vi "Relay Experiment V2 - Ramps.vi"() -> ()   [LabVIEW 2020]
uses:
  <vilib>/Analysis/1siggen.llb/Ramp Pattern by Samples.vi
  <vilib>/DAQmx/write.llb/DAQmx Write (Analog 1D Wfm NChan NSamp).vi
  <vilib>/DAQmx/create/channels.llb/DAQmx Create Channel (AO-Voltage-Basic).vi
  <vilib>/DAQmx/configure/timing.llb/DAQmx Timing (Use Waveform).vi
  <vilib>/DAQmx/miscellaneous.llb/DAQmx Fill In Error Info.vi
  <vilib>/Analysis/NI_AALBase.lvlib
  <vilib>/measure/NI_MABase.lvlib
panel:
  in  "Trigger 2 Channel":tag="Dev2/ao3"
  in  "AC Output Channel":tag="Dev2/ao1"
  in  "Trigger 1 Channel":tag="Dev2/ao2"
  in  "DC Output Channel":tag="Dev2/ao0"
  out "DC Sampling\nFrequency (Hz)":dbl
  in  "Stop":bool
  in  "DC-to-AC\nDelay Time (ms)":dbl min=0.0 step=1.0
  in  "Trailing Pulse\nRamp Time (ms)":dbl=200.0 min=0.0
  in  "Leading Pulse\nRamp Time (ms)":dbl=200.0 min=0.0
  in  "AC Source\nGain":dbl=5.0
  out "DC On":bool=TRUE
  out "AC On":bool
  in  "Waveform Type":u16(ring) items=["Sine Wave", "Triangle Wave", "Square Wave", "Sawtooth Wave"]
  out "DC Waveform Graph":waveform(dbl)(graph)
  in  "AC  Waveform\nFrequency (Hz)":i32=20000 min=0 max=100000 step=10
  out "DC Total\nTime (s)":dbl
  in  "DC Recharge\nRamp Time (s)":dbl=1.0 min=0.0
  in  "AC  Waveform\nAmplitude\n(Vpp/mApp)":dbl
  out "DC Recharge\nTime (s)":dbl
  out "DC Pulse\nCharge (mC)":dbl
  in  "DC Recharge\nAmplitude (mA)":dbl=0.1 min=1e-06
  in  "DC Pulse\nAmplitude (mA)":dbl=-1.0 max=-1e-06
  in  "DC Pulse\nPlateau Time (ms)":dbl=100.0 min=0.0
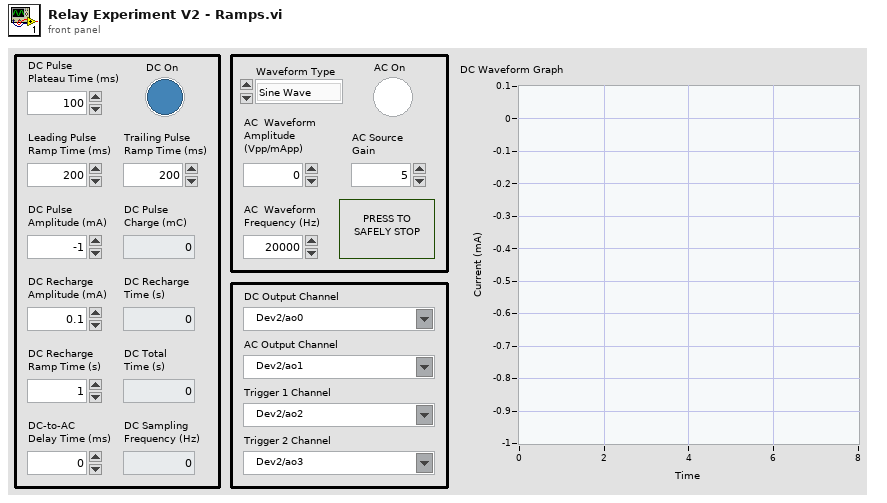
[diagram p1: front panel]
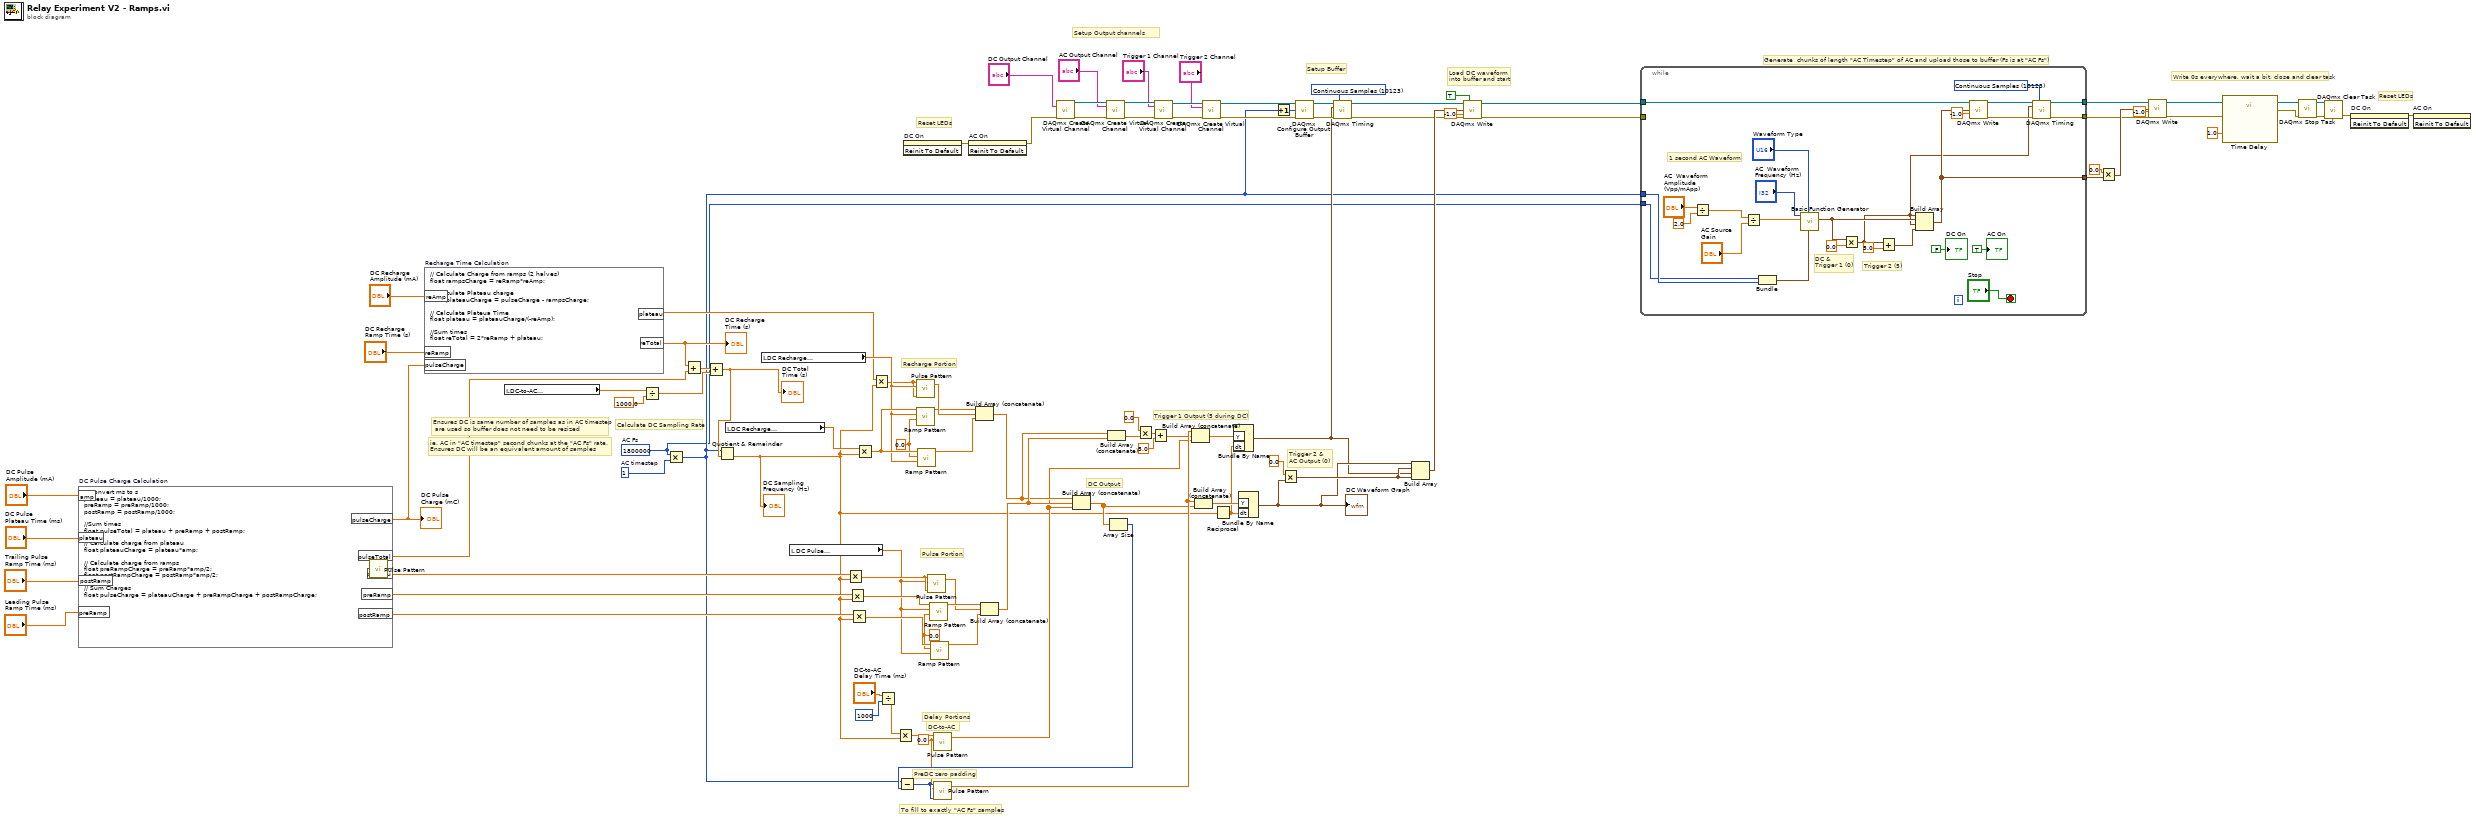
[diagram p0: block diagram]
diagram:
  w6 = 1  # AC timestep
  w44 = 10123 items=["Finite Samples"=10178, "Continuous Samples"=10123, "Hardware Timed Single Point"=12522] ("sample mode")
  w4 = 1800000  # AC Fs
  w67 = 0.0 ("amplitude")
  w80 = 0.0 ("start")
  w90 = 0.0 ("end")
  # "Reset LEDs"
  # "Reset LEDs"
  # "Write 0s everywhere, wait a bit, close and clear task"
  # "Generate  chunks of length \"AC Timestep\" of AC and upload those to buffer (Fs is at \"AC Fs\")"
  # "Load DC waveform\ninto buffer and start"
  # "Setup Buffer"
  # "Trigger 1 Output (5 during DC)"
  # "Trigger 2 &\nAC Output (0)"
  # "DC Output"
  # "Setup Output channels"
  # "ie. AC in \"AC timestep\" second chunks at the \"AC Fs\" rate.  \nEnsures DC will be an equivalent amount of samples"
  # "To fill to exactly \"AC Fs\" samples"
  # "PreDC zero padding"
  # "DC-to-AC"
  # "Ensures DC is same number of samples as in AC timestep\n are used so buffer does not need to be resized"
  # "Calculate DC Sampling Rate"
  # "Delay Portions"
  # "Pulse Portion"
  # "Recharge Portion"
  n1 = formula code="// Convert ms to s\nplateau = plateau/1000;\npreRamp = preRamp/1000;\npostRamp = postRamp/1000;\n\n//Sum times\nfloat pulseTotal = plateau + preRamp + postRamp;\n\n// Calculate charge from plateau\nfloat plateauCharge = plateau*amp;\n\n// Calculate charge from ramps\nfloat preRampCharge = preRamp*amp/2;\nfloat postRampCharge = postRamp*amp/2;\n\n// Sum Charges\nfloat pulseCharge = plateauCharge + preRampCharge + postRampCharge;" "DC Pulse Charge Calculation"("amp"="DC Pulse\nAmplitude (mA)", "plateau"="DC Pulse\nPlateau Time (ms)", "postRamp"="Trailing Pulse\nRamp Time (ms)", "preRamp"="Leading Pulse\nRamp Time (ms)") -> ("pulseCharge"=w97:dbl, "pulseTotal"=w93:dbl, "plateau"=w86:dbl, "preRamp"=w85:dbl, "postRamp"=w84:dbl)
  "DC Pulse\nCharge (mC)" <- w97
  n2 = call <vilib>:"Pulse Pattern.vi"() -> ()  [unwired: 4 in, 2 out]
  n3 = formula code="// Calculate Charge from ramps (2 halves)\nfloat rampsCharge = reRamp*reAmp;\n\n// Calculate Plateau charge\nfloat plateauCharge = pulseCharge - rampsCharge;\n\n// Calculate Plateua Time\nfloat plateau = plateauCharge/(-reAmp);\n\n//Sum times\nfloat reTotal = 2*reRamp + plateau;" "Recharge Time Calculation"("pulseCharge"=w97, "reRamp"="DC Recharge\nRamp Time (s)", "reAmp"="DC Recharge\nAmplitude (mA)") -> ("plateau"=w88:dbl, "reTotal"=w94:dbl)
  "DC Recharge\nTime (s)" <- w94
  n4 = local read "DC-to-AC\nDelay Time (ms)"() -> (w3:dbl)
  n5 = Divide(x=w3, y=1000.0) -> (x/y=w7:dbl)
  n6 = Multiply(x=w4, y=w6) -> (x*y=w5:i32)
  n7 = Add(x=w94, y=w93) -> (x+y=w11:dbl)
  n8 = Add(x=w11, y=w7) -> (x+y=w10:dbl)
  "DC Total\nTime (s)" <- w10
  n9 = Quotient & Remainder(x=w5, y=w10) -> (floor(x/y)=w9:dbl)  [unwired: 1 out]
  "DC Sampling\nFrequency (Hz)" <- w9
  n10 = local read "DC Recharge\nRamp Time (s)"() -> (w92:dbl)
  n11 = local read "DC Recharge\nAmplitude (mA)"() -> (w89:dbl)
  n12 = local read "DC Pulse\nAmplitude (mA)"() -> (w79:dbl)
  n13 = Multiply(x=w86, y=w9) -> (x*y=w83:dbl)
  n14 = Multiply(x=w85, y=w9) -> (x*y=w82:dbl)
  n15 = Multiply(x=w84, y=w9) -> (x*y=w81:dbl)
  n16 = Multiply(x=w92, y=w9) -> (x*y=w91:dbl)
  n17 = Multiply(x=w88, y=w9) -> (x*y=w87:dbl)
  n18 = Divide(x="DC-to-AC\nDelay Time (ms)", y=1000) -> (x/y=w70:dbl)
  n19 = Multiply(x=w70, y=w9) -> (x*y=w72:dbl)
  n20 = invoke on="DC On" class="Bool (strict)" method="Reinit To Default"() -> (error out=w25:errorcluster)  [unwired: 3 in, 2 out]
  n21 = call <vilib>:"Pulse Pattern.vi"("width"=w87, "amplitude"=w89, "samples"=w87) -> ("Pulse Pattern"=w78:dbl[])  [unwired: 1 in, 1 out]
  n22 = call-poly <vilib>:"Ramp Pattern.vi"("start"=w90, "end"=w89, "samples"=w91) -> ("Ramp Pattern"=w77:dbl[])  [unwired: 7 in, 1 out]
  n23 = call-poly <vilib>:"Ramp Pattern.vi"("start"=w89, "end"=w90, "samples"=w91) -> ("Ramp Pattern"=w76:dbl[])  [unwired: 7 in, 1 out]
  n24 = call <vilib>:"Pulse Pattern.vi"("width"=w83, "amplitude"=w79, "samples"=w83) -> ("Pulse Pattern"=w74:dbl[])  [unwired: 1 in, 1 out]
  n25 = call-poly <vilib>:"Ramp Pattern.vi"("start"=w80, "end"=w79, "samples"=w82) -> ("Ramp Pattern"=w75:dbl[])  [unwired: 7 in, 1 out]
  n26 = call-poly <vilib>:"Ramp Pattern.vi"("start"=w79, "end"=w80, "samples"=w81) -> ("Ramp Pattern"=w73:dbl[])  [unwired: 7 in, 1 out]
  n27 = call <vilib>:"Pulse Pattern.vi"("amplitude"=w67, "samples"=w72) -> ("Pulse Pattern"=w46:dbl[])  [unwired: 2 in, 1 out]
  n28 = invoke on="AC On" class="Bool (strict)" method="Reinit To Default"(error in=w25) -> (error out=w24:errorcluster)  [unwired: 2 in, 2 out]
  n29 = Build Array (concatenate)(w77, w78, w76) -> (w49:dbl[])
  n30 = Build Array (concatenate)(w75, w74, w73) -> (w50:dbl[])
  n31 = call-poly <vilib>:"DAQmx Create Virtual Channel.vi"("physical channels"="DC Output Channel", "error in"=w24) -> ("task out"=w63:refnum<k21>, "error out"=w64:errorcluster)  [unwired: 12 in]
  n32 = Build Array (concatenate)(w49, w50, w46) -> (w12:dbl[])
  n33 = call-poly <vilib>:"DAQmx Create Virtual Channel.vi"("task in"=w63, "physical channels"="AC Output Channel", "error in"=w64) -> ("task out"=w60:refnum<k21>, "error out"=w61:errorcluster)  [unwired: 11 in]
  n34 = Build Array (concatenate)(w49, w50) -> (w48:dbl[])
  n35 = Array Size(array=w12) -> (size(s)=w69:i32)
  n36 = Subtract(x=w5, y=w69) -> (x-y=w68:i32)
  n37 = call <vilib>:"Pulse Pattern.vi"("width"=w68, "amplitude"=w67, "samples"=w68) -> ("Pulse Pattern"=w47:dbl[])  [unwired: 1 in, 1 out]
  n38 = Multiply(x=0.0 ("amplitude"), y=w48) -> (x*y=w51:dbl[])
  n39 = Add(x=w51, y=5.0) -> (x+y=w18:dbl[])
  n40 = call-poly <vilib>:"DAQmx Create Virtual Channel.vi"("task in"=w60, "physical channels"="Trigger 1 Channel", "error in"=w61) -> ("task out"=w57:refnum<k21>, "error out"=w58:errorcluster)  [unwired: 11 in]
  n41 = Build Array (concatenate)(w47, w18, w46) -> (w13:dbl[])
  n42 = Build Array (concatenate)(w47, w12) -> (w66:dbl[])
  n43 = call-poly <vilib>:"DAQmx Create Virtual Channel.vi"("task in"=w57, "physical channels"="Trigger 2 Channel", "error in"=w58) -> ("task out"=w55:refnum<k21>, "error out"=w27:errorcluster)  [unwired: 11 in]
  n44 = Reciprocal(x=w9) -> (1/x=w45:dbl)
  n45 = Bundle By Name("Y"=w13, "dt"=w45) -> (w14:waveform(dbl))  [unwired: 1 in]
  n46 = Bundle By Name("Y"=w66, "dt"=w45) -> (w41:waveform(dbl))  [unwired: 1 in]
  "DC Waveform Graph" <- w41
  n47 = Increment(x=w5) -> (x+1=w15:i32)
  n48 = Multiply(x=0.0 ("amplitude"), y=w41) -> (x*y=w42:waveform(dbl))
  n49 = call <vilib>:"DAQmx Configure Output Buffer.vi"("task/channels in"=w55, "buffer size (in samples per channel)"=w15, "error in"=w27) -> ("task out"=w43:refnum<k21>, "error out"=w26:errorcluster)  [unwired: 11 in]
  n50 = call-poly <vilib>:"DAQmx Timing.vi"("task/channels in"=w43, "sample mode"=w44, "waveform"=w14, "error in"=w26) -> ("task out"=w40:refnum<k21>, "error out"=w17:errorcluster)  [unwired: 10 in]
  n51 = Build Array(w41, w42, w14, w42) -> (w38:waveform(dbl)[])
  n52 = call-poly <vilib>:"DAQmx Write.vi"("task/channels in"=w40, "auto start"=TRUE, "data"=w38, "timeout"=-1.0, "error in"=w17) -> ("task out"=w16:refnum<k21>, "error out"=w1:errorcluster)  [unwired: 8 in, 1 out]
  n53 = while {
    tunnel: w5 -> [w103]
    tunnel: w16 -> [w110]
    tunnel: [w107] -> w35
    tunnel: [w111] -> w36
    tunnel: [w108] -> w21
    tunnel: w4 -> [w102]
    tunnel: w1 -> [_]
    stop <- "Stop" stop-if-true
    w104 = 10123 items=["Finite Samples"=10178, "Continuous Samples"=10123, "Hardware Timed Single Point"=12522] ("sample mode")
    # "1 second AC Waveform"
    # "Trigger 2 (5)"
    # "DC &\nTrigger 1 (0)"
    n54 = Divide(x="AC  Waveform\nAmplitude\n(Vpp/mApp)", y=2.0) -> (x/y=w123:dbl)
    n55 = Divide(x=w123, y="AC Source\nGain") -> (x/y=w121:dbl)
    n56 = Bundle("AC Fs"=w102, w103) -> (w117:cluster{"AC Fs":i32, i32})  [unwired: 1 in]
    n57 = call <vilib>:"Basic Function Generator.vi"("sampling info"=w117, "signal type"="Waveform Type", "amplitude"=w121, "frequency"="AC  Waveform\nFrequency (Hz)") -> ("signal out"=w113:waveform(dbl))  [unwired: 5 in, 2 out]
    n58 = Multiply(x=w113, y=0.0 ("x")) -> (x*y=w105:waveform(dbl))
    n59 = Add(x=w105, y=5.0) -> (x+y=w112:waveform(dbl))
    n60 = Build Array(w105, w113, w105, w112) -> (w111:waveform(dbl)[])
    n61 = call-poly <vilib>:"DAQmx Write.vi"("task/channels in"=w110, "data"=w111, "timeout"=-1.0) -> ("task out"=w106:refnum<k21>, "error out"=w109:errorcluster)  [unwired: 10 in, 1 out]
    n62 = call-poly <vilib>:"DAQmx Timing.vi"("task/channels in"=w106, "sample mode"=w104, "waveform"=w105, "error in"=w109) -> ("task out"=w107:refnum<k21>, "error out"=w108:errorcluster)  [unwired: 10 in]
    "AC On" <- TRUE ("AC On")
    "DC On" <- FALSE ("DC On")
  }
  n63 = Multiply(x=0.0, y=w36) -> (x*y=w34:waveform(dbl)[])
  n64 = call-poly <vilib>:"DAQmx Write.vi"("task/channels in"=w35, "data"=w34, "timeout"=-1.0, "error in"=w21) -> ("task out"=w31:refnum<k21>, "error out"=w20:errorcluster)  [unwired: 9 in, 1 out]
  n65 = call "Time Delay"("error in (no error)"=w20, "Delay Time (s)"=1.0) -> ("error out"=w30:errorcluster)  [unwired: 9 in]
  n66 = call <vilib>:"DAQmx Stop Task.vi"("task/channels in"=w31, "error in"=w30) -> ("task out"=w29:refnum<k21>, "error out"=w28:errorcluster)  [unwired: 12 in]
  n67 = call <vilib>:"DAQmx Clear Task.vi"("task in"=w29, "error in"=w28) -> ("error out"=w22:errorcluster)  [unwired: 13 in]
  n68 = invoke on="DC On" class="Bool (strict)" method="Reinit To Default"(error in=w22) -> (error out=w23:errorcluster)  [unwired: 2 in, 2 out]
  n69 = invoke on="AC On" class="Bool (strict)" method="Reinit To Default"(error in=w23) -> ()  [unwired: 2 in, 3 out]
